vi "FTW-JSON-Core-GetFlattenedValue.vi"(0 "Container":refnum<class "FTW-Container.lvclass">, 7 "LabVIEW Type":T1, 9 "Element Default Value":variant, 11 "error in":errorcluster, 12 "Encoding Flags":i64 format="%016x") -> (4 "Flattened Value":string, 15 "error out":errorcluster)   [LabVIEW 2015]
uses:
  Reflection/FTW-Reflection-Types.ctl
  container/FTW-Container.lvclass
  Error/FTW-ERR-ThrowError.vi
panel:
  # "Inputs"
  # "Outputs"
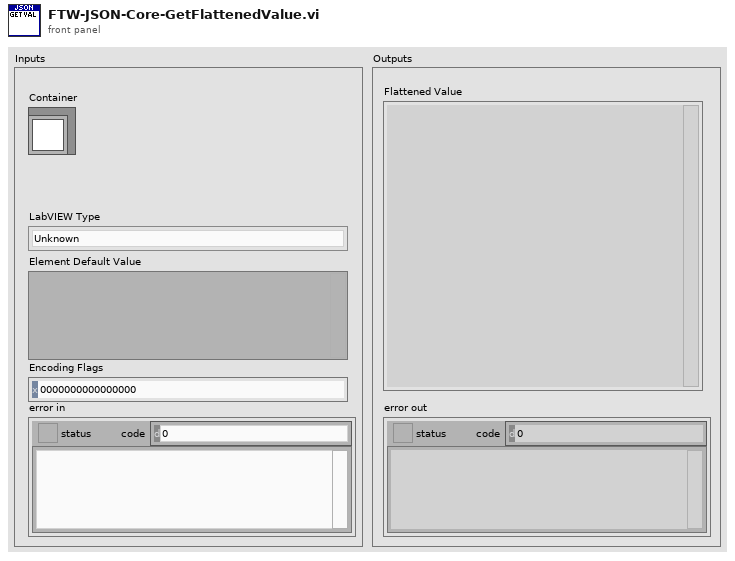
[diagram p1: front panel]
types:
  T1 = typedef "FTW-Reflection-Types.ctl" = enum16{"Unknown", "Void", "Array", "Cluster", "LVObject", "Boolean", "I8", "I16", "I32", "I64", "U8", "U16", "U32", "U64", "SGL", "DBL", "EXT", "CSG", "CDB", "CXT", "FXP", "EnumU8", "EnumU16", "EnumU32", "EnumU64", "SGLwithUnit", "DBLwithUnit", "EXTwithUnit", "CSGwithUnit", "CDBwithUnit", "CXTwithUnit", "String", "Path", "Picture", "Tag", "LVVariant", "Timestamp", "WaveformI8", "WaveformI16", "WaveformI32", "WaveformI64", "WaveformU8", "WaveformU16", "WaveformU32", "WaveformU64", "WaveformSGL", "WaveformDBL", "WaveformEXT", "WaveformCSG", "WaveformCDB", "WaveformCXT", "WaveformDigital", "WaveformUnknownType", "DigitalData", "DynamicData", "ExternalData", "FileByteStream", "TDMStream", "dotNET", "ActiveX", "VIServerReference", "VIReference", "ApplicationInstance", "Menu", "ConnectionDataSocket", "ConnectionVISA", "ConnectionBluetooth", "ConnectionIrDA", "ConnectionTCP", "ConnectionUDP", "ConnectionHTTPClient", "ConnectionFTP", "Occurrence", "Notifier", "Queue", "Rendezvous", "Semaphore", "RTFIFO", "EventPublisher", "EventRegistration", "EventCallback", "DataValueReference", "GenericClass", "GenericClassTag", "GenericClassDeepCopy", "GenericClassFlattened", "GenericClassTagFlattened", "GenericReferenceType", "WindowsRegistry", "OverloadedDatalogRef", "ReferenceUnknownType"}
  T2 = typedef "NI_Data Type.lvlib/Data Type.ctl" = enum8{"Invalid Type", "Void", "I8", "I16", "I32", "I64", "U8", "U16", "U32", "U64", "Single Float", "Double Float", "Extended Float", "Single Complex", "Double Complex", "Extended Complex", "Enum U8", "Enum U16", "Enum U32", "Enum U64", "Single Float With Unit", "Double Float With Unit", "Extended Float With Unit", "Single Complex with Unit", "Double Complex with Unit", "Extended Complex with Unit", "Boolean", "String", "Path", "Picture", "Tag", "Array", "Cluster", "Variant", "LV Variant", "Waveform", "Timestamp", "Digital Waveform", "Digital Data", "ExpressData", "Refnum", "External Data", "VI", "Poly VI", "LabVIEW Class Instance", "Fixed Point"}
  T3 = cluster{"Element Name":string, "Element Type":T1, "Element Value":variant}[]
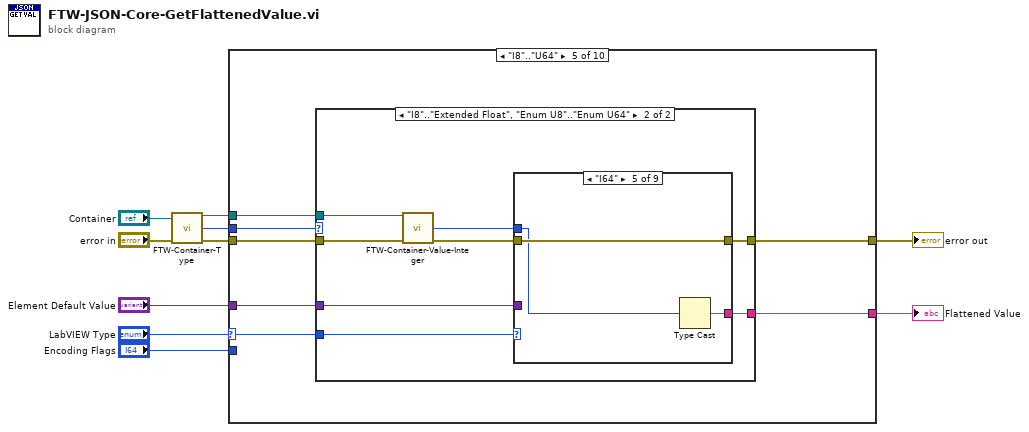
[diagram p0: block diagram]
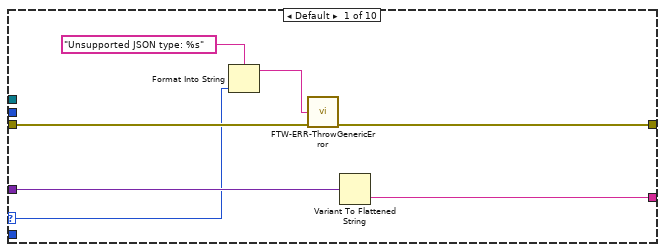
[diagram p2: hidden frame]
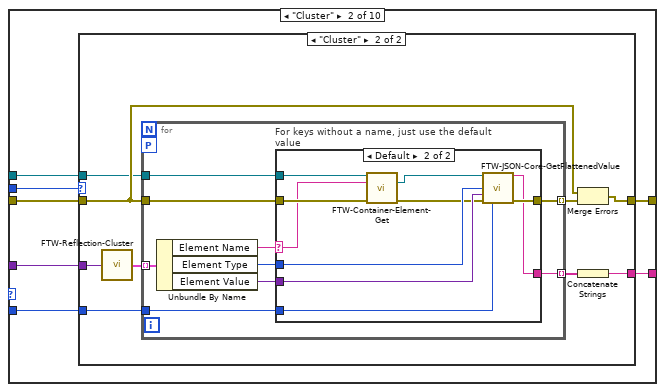
[diagram p3: hidden frame]
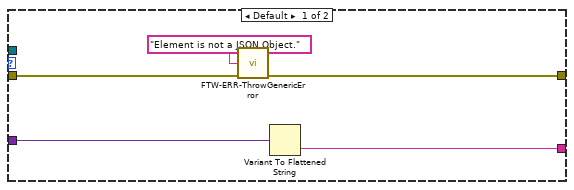
[diagram p4: hidden frame]
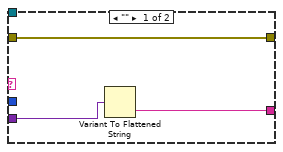
[diagram p5: hidden frame]
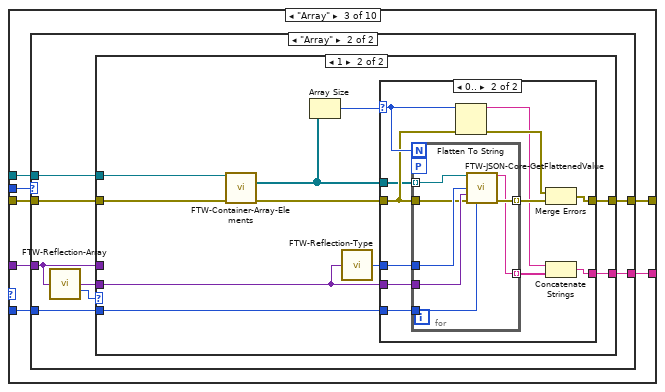
[diagram p6: hidden frame]
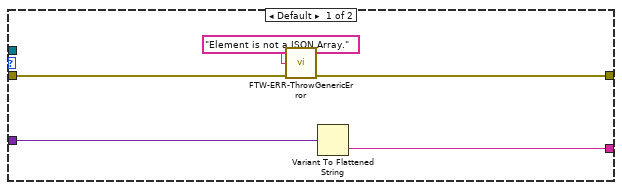
[diagram p7: hidden frame]
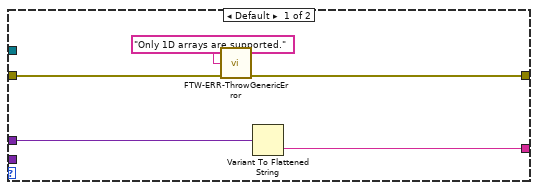
[diagram p8: hidden frame]
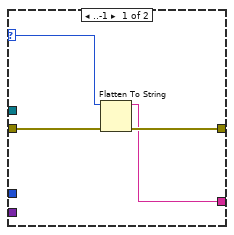
[diagram p9: hidden frame]
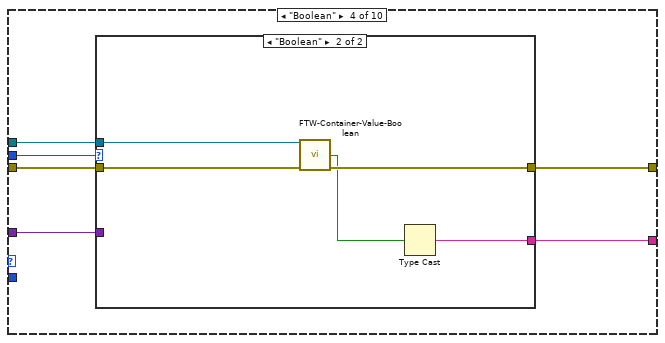
[diagram p10: hidden frame]
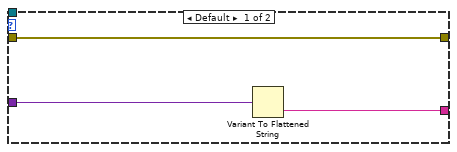
[diagram p11: hidden frame]
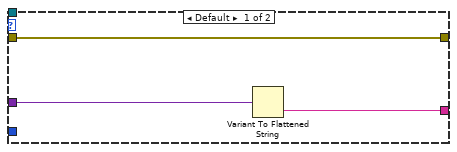
[diagram p12: hidden frame]
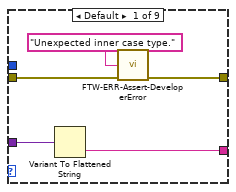
[diagram p13: hidden frame]
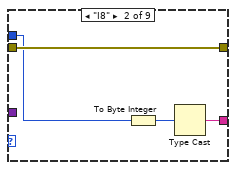
[diagram p14: hidden frame]
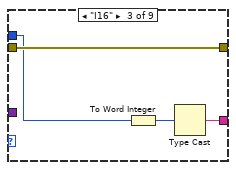
[diagram p15: hidden frame]
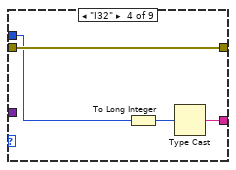
[diagram p16: hidden frame]
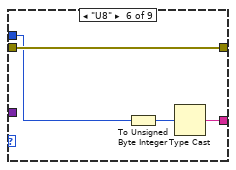
[diagram p17: hidden frame]
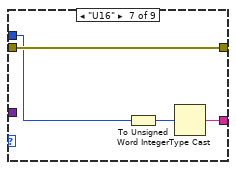
[diagram p18: hidden frame]
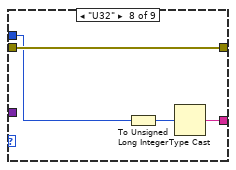
[diagram p19: hidden frame]
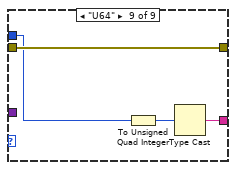
[diagram p20: hidden frame]
diagram:
  n1 = call "FTW-Container-Type.vi"("FTW-Container In"="Container", "error in"="error in") -> ("FTW-Container Out"=w2:refnum<class "FTW-Container.lvclass">, "Type"=w1:T2, "error out"=w4:errorcluster)  [unwired: 11 in]
  n2 = case shown="\"I8\"..\"U64\"" "LabVIEW Type" {
    selector: "LabVIEW Type" -> [w11 _ _ _ w136 w190 w260 _ w319 _]
    tunnel: [w14 w22 w65 w120 w134 w188 w258 w292 w317 w363] -> w10
    tunnel: [w12 w23 w66 w123 w138 w192 w262 w295 w321 w366] -> w8
    tunnel: w4 -> [w15 w21 w64 w124 w139 w193 w263 w296 w322 w367]
    tunnel: "Element Default Value" -> [w13 w24 w67 w122 w137 w191 w261 w294 w320 w365]
    tunnel: w1 -> [_ w20 w63 w121 w135 w189 w259 w293 w318 w364]
    tunnel: "Encoding Flags" -> [_ w19 w62 _ _ _ _ _ w316 _]
    tunnel: w2 -> [_ w18 w61 w119 w133 w187 w257 w291 w315 w362]
    frame Default {
      n3 = Format Into String(format string="Unsupported JSON type: %s", w11) -> (resulting string=w17:string)  [unwired: 2 in, 1 out]
      n4 = call "FTW-ERR-ThrowGenericError.vi"("Error Message"=w17, "error in"=w15) -> ("error out"=w14:errorcluster)  [unwired: 13 in]
      n5 = Variant To Flattened String(Variant=w13) -> (data string=w12:string)  [unwired: 1 out]
    }
    frame "Cluster" {
      n6 = case shown="\"Cluster\"" w20 {
        tunnel: w24 -> [w27 w38]
        tunnel: [w26 w37] -> w23
        tunnel: [w28 w36] -> w22
        tunnel: w21 -> [w29 w31]
        tunnel: w19 -> [_ w35]
        tunnel: w18 -> [_ w30]
        frame Default {
          n7 = call "FTW-ERR-ThrowGenericError.vi"("Error Message"="Element is not a JSON Object.", "error in"=w29) -> ("error out"=w28:errorcluster)  [unwired: 13 in]
          n8 = Variant To Flattened String(Variant=w27) -> (data string=w26:string)  [unwired: 1 out]
        }
        frame "Cluster" {
          n9 = call "FTW-Reflection-Cluster.vi"("Cluster"=w38) -> ("Cluster Elements"=w34:T3)  [unwired: 14 in]
          n10 = for {
            tunnel: w34 -> [w46] mode=indexing
            tunnel: [w44] -> w33 mode=indexing
            tunnel: w31 -> [w47]
            tunnel: [w42] -> w32 mode=indexing
            workers-P: _ -> [_]
            tunnel: w35 -> [w41]
            tunnel: w30 -> [w39]
            n11 = Unbundle By Name(w46) -> ("Element Name"=w40:string, "Element Type"=w43:T1, "Element Value"=w45:variant)
            n12 = case "For keys without a name, just use the default value" shown="Default" w40 {
              selector: w40 -> [_ w52]
              tunnel: w47 -> [w48 w60]
              tunnel: w45 -> [w50 w57]
              tunnel: [w49 w58] -> w44
              tunnel: w43 -> [_ w56]
              tunnel: [w48 w59] -> w42
              tunnel: w41 -> [_ w55]
              tunnel: w39 -> [_ w53]
              frame "" {
                n13 = Variant To Flattened String(Variant=w50) -> (data string=w49:string)  [unwired: 1 out]
              }
              frame Default {
                n14 = call "FTW-Container-Element-Get.vi"("FTW-Container In"=w53, "Element Name"=w52, "error in"=w60) -> ("Element Out"=w51:refnum<class "FTW-Container.lvclass">, "error out"=w54:errorcluster)  [unwired: 9 in, 2 out]
                n15 = call "FTW-JSON-Core-GetFlattenedValue.vi"("Container"=w51, "LabVIEW Type"=w56, "Element Default Value"=w57, "error in"=w54, "Encoding Flags"=w55) -> ("Flattened Value"=w58:string, "error out"=w59:errorcluster)  [unwired: 9 in]
              }
            }
          }
          n16 = Merge Errors(w31, w32) -> (w36:errorcluster)
          n17 = Concatenate Strings(w33) -> (w37:string)
        }
      }
    }
    frame "Array" {
      n18 = case shown="\"Array\"" w63 {
        tunnel: w67 -> [w70 w75]
        tunnel: [w69 w80] -> w66
        tunnel: [w68 w79] -> w65
        tunnel: w64 -> [w71 w78]
        tunnel: w62 -> [_ w74]
        tunnel: w61 -> [_ w73]
        frame Default {
          n19 = call "FTW-ERR-ThrowGenericError.vi"("Error Message"="Element is not a JSON Array.", "error in"=w71) -> ("error out"=w68:errorcluster)  [unwired: 13 in]
          n20 = Variant To Flattened String(Variant=w70) -> (data string=w69:string)  [unwired: 1 out]
        }
        frame "Array" {
          n21 = call "FTW-Reflection-Array.vi"("Array"=w75) -> ("Default Array Element"=w77:variant, "Number of Dimensions"=w76:i32)  [unwired: 13 in]
          n22 = case shown="1" w76 {
            tunnel: [w82 w95] -> w80
            tunnel: [w83 w94] -> w79
            tunnel: w78 -> [w84 w91]
            tunnel: w77 -> [_ w90]
            tunnel: w75 -> [w81 _]
            tunnel: w74 -> [_ w92]
            tunnel: w73 -> [_ w88]
            frame Default {
              n23 = call "FTW-ERR-ThrowGenericError.vi"("Error Message"="Only 1D arrays are supported.", "error in"=w84) -> ("error out"=w83:errorcluster)  [unwired: 13 in]
              n24 = Variant To Flattened String(Variant=w81) -> (data string=w82:string)  [unwired: 1 out]
            }
            frame 1 {
              n25 = call "FTW-Container-Array-Elements.vi"("FTW-Container In"=w88, "error in"=w91) -> ("Array Elements"=w86:refnum<class "FTW-Container.lvclass">[], "error out"=w89:errorcluster)  [unwired: 11 in, 1 out]
              n26 = Array Size(array=w86) -> (size(s)=w87:i32)
              n27 = call "FTW-Reflection-Type.vi"("Anything"=w90) -> ("LabVIEW Type"=w93:T1)  [unwired: 12 in, 2 out]
              n28 = case shown="0.." w87 {
                selector: w87 -> [w97 w105]
                tunnel: [w96 w111] -> w95
                tunnel: [w98 w110] -> w94
                tunnel: w89 -> [w99 w102]
                tunnel: w93 -> [_ w108]
                tunnel: w90 -> [_ w107]
                tunnel: w92 -> [_ w101]
                tunnel: w86 -> [_ w100]
                frame ..-1 {
                  n29 = Flatten To String(anything=w97, error in (no error)=w99) -> (data string=w96:string, error out=w98:errorcluster)  [unwired: 2 in, 1 out]
                }
                frame 0.. {
                  n30 = for {
                    N: w105 -> [_]
                    workers-P: _ -> [_]
                    tunnel: w102 -> [w113]
                    tunnel: [w118] -> w109 mode=indexing
                    tunnel: w108 -> [w115]
                    tunnel: w107 -> [w116]
                    tunnel: [w117] -> w106 mode=indexing
                    tunnel: w101 -> [w114]
                    tunnel: w100 -> [w112] mode=indexing
                    n31 = call "FTW-JSON-Core-GetFlattenedValue.vi"("Container"=w112, "LabVIEW Type"=w115, "Element Default Value"=w116, "error in"=w113, "Encoding Flags"=w114) -> ("Flattened Value"=w117:string, "error out"=w118:errorcluster)  [unwired: 9 in]
                  }
                  n32 = Flatten To String(anything=w105, error in (no error)=w102) -> (data string=w103:string, error out=w104:errorcluster)  [unwired: 2 in, 1 out]
                  n33 = Merge Errors(w104, w109) -> (w110:errorcluster)
                  n34 = Concatenate Strings(w103, w106) -> (w111:string)
                }
              }
            }
          }
        }
      }
    }
    frame "Boolean" {
      n35 = case shown="\"Boolean\"" w121 {
        tunnel: w124 -> [w125 w131]
        tunnel: w122 -> [w127 _]
        tunnel: [w126 w132] -> w123
        tunnel: [w125 w130] -> w120
        tunnel: w119 -> [_ w129]
        frame Default {
          n36 = Variant To Flattened String(Variant=w127) -> (data string=w126:string)  [unwired: 1 out]
        }
        frame "Boolean" {
          n37 = call "FTW-Container-Value-Boolean.vi"("FTW-Container In"=w129, "error in"=w131) -> ("Value"=w128:bool, "error out"=w130:errorcluster)  [unwired: 11 in, 1 out]
          n38 = Type Cast(x=w128) -> (*(type *) &x=w132:string)  [unwired: 1 in]
        }
      }
    }
    frame "I8".."U64" {
      n39 = case shown="\"I8\"..\"Extended Float\", \"Enum U8\"..\"Enum U64\"" w135 {
        tunnel: w139 -> [w140 w148]
        tunnel: w137 -> [w142 w146]
        tunnel: [w141 w147] -> w138
        tunnel: [w140 w149] -> w134
        tunnel: w136 -> [_ w150]
        tunnel: w133 -> [_ w144]
        frame Default {
          n40 = Variant To Flattened String(Variant=w142) -> (data string=w141:string)  [unwired: 1 out]
        }
        frame "I8".."Extended Float", "Enum U8".."Enum U64" {
          n41 = call "FTW-Container-Value-Integer.vi"("JSON"=w144, "error in"=w148) -> ("Value"=w143:i64, "error out"=w145:errorcluster)  [unwired: 11 in, 1 out]
          n42 = case shown="\"I64\"" w150 {
            tunnel: [w154 w159 w163 w167 w170 w174 w178 w182 w186] -> w149
            tunnel: w145 -> [w155 w159 w163 w167 w170 w174 w178 w182 w186]
            tunnel: w143 -> [_ w157 w161 w165 w168 w172 w176 w180 w184]
            tunnel: [w151 w158 w162 w166 w169 w173 w177 w181 w185] -> w147
            tunnel: w146 -> [w152 _ _ _ _ _ _ _ _]
            frame Default {
              n43 = Variant To Flattened String(Variant=w152) -> (data string=w151:string)  [unwired: 1 out]
              n44 = call "FTW-ERR-Assert-DeveloperError.vi"("Reason this error should never happen"="Unexpected inner case type.", "error in"=w155) -> ("error out"=w154:errorcluster)  [unwired: 13 in]
            }
            frame "I8" {
              n45 = To Byte Integer(number=w157) -> (8bit integer=w156:i8)
              n46 = Type Cast(x=w156) -> (*(type *) &x=w158:string)  [unwired: 1 in]
            }
            frame "I16" {
              n47 = To Word Integer(number=w161) -> (16bit integer=w160:i16)
              n48 = Type Cast(x=w160) -> (*(type *) &x=w162:string)  [unwired: 1 in]
            }
            frame "I32" {
              n49 = To Long Integer(number=w165) -> (32bit integer=w164:i32)
              n50 = Type Cast(x=w164) -> (*(type *) &x=w166:string)  [unwired: 1 in]
            }
            frame "I64" {
              n51 = Type Cast(x=w168) -> (*(type *) &x=w169:string)  [unwired: 1 in]
            }
            frame "U8" {
              n52 = To Unsigned Byte Integer(number=w172) -> (unsigned 8bit integer=w171:u8)
              n53 = Type Cast(x=w171) -> (*(type *) &x=w173:string)  [unwired: 1 in]
            }
            frame "U16" {
              n54 = To Unsigned Word Integer(number=w176) -> (unsigned 16bit integer=w175:u16)
              n55 = Type Cast(x=w175) -> (*(type *) &x=w177:string)  [unwired: 1 in]
            }
            frame "U32" {
              n56 = To Unsigned Long Integer(number=w180) -> (unsigned 32bit integer=w179:u32)
              n57 = Type Cast(x=w179) -> (*(type *) &x=w181:string)  [unwired: 1 in]
            }
            frame "U64" {
              n58 = To Unsigned Quad Integer(1:w184) -> (0:w183:u64)
              n59 = Type Cast(x=w183) -> (*(type *) &x=w185:string)  [unwired: 1 in]
            }
          }
        }
      }
    }
    frame "EnumU8".."EnumU64" {
      n60 = case shown="\"String\"" w189 {
        tunnel: w193 -> [w194 w206 w231]
        tunnel: w191 -> [w196 w200 w235]
        tunnel: [w195 w203 w232] -> w192
        tunnel: [w194 w204 w233] -> w188
        tunnel: w190 -> [_ w205 w234]
        tunnel: w187 -> [_ w198 w229]
        frame Default {
          n61 = Variant To Flattened String(Variant=w196) -> (data string=w195:string)  [unwired: 1 out]
        }
        frame "String" {
          n62 = call "FTW-Container-Value-String.vi"("JSON"=w198, "error in"=w206) -> ("Value"=w197:string, "error out"=w199:errorcluster)  [unwired: 11 in, 1 out]
          n63 = call "FTW-Reflection-Enum.vi"("Enum"=w200) -> ("Enum Items"=w202:string[])  [unwired: 12 in, 2 out]
          n64 = Search 1D Array(1D array=w202, element=w197) -> (index of element=w201:i32)  [unwired: 1 in]
          n65 = case shown="\"EnumU8\"" w205 {
            tunnel: [w210 w215 w219 w223 w227] -> w204
            tunnel: w199 -> [w211 w215 w219 w223 w227]
            tunnel: [w208 w214 w218 w222 w226] -> w203
            tunnel: w201 -> [_ w212 w216 w220 w224]
            tunnel: w200 -> [w207 _ _ _ _]
            frame Default {
              n66 = Variant To Flattened String(Variant=w207) -> (data string=w208:string)  [unwired: 1 out]
              n67 = call "FTW-ERR-Assert-DeveloperError.vi"("Reason this error should never happen"="Unexpected inner case type.", "error in"=w211) -> ("error out"=w210:errorcluster)  [unwired: 13 in]
            }
            frame "EnumU8" {
              n68 = To Unsigned Byte Integer(number=w212) -> (unsigned 8bit integer=w213:u8)
              n69 = Type Cast(x=w213) -> (*(type *) &x=w214:string)  [unwired: 1 in]
            }
            frame "EnumU16" {
              n70 = To Unsigned Word Integer(number=w216) -> (unsigned 16bit integer=w217:u16)
              n71 = Type Cast(x=w217) -> (*(type *) &x=w218:string)  [unwired: 1 in]
            }
            frame "EnumU32" {
              n72 = To Unsigned Long Integer(number=w220) -> (unsigned 32bit integer=w221:u32)
              n73 = Type Cast(x=w221) -> (*(type *) &x=w222:string)  [unwired: 1 in]
            }
            frame "EnumU64" {
              n74 = To Unsigned Quad Integer(1:w224) -> (0:w225:u64)
              n75 = Type Cast(x=w225) -> (*(type *) &x=w226:string)  [unwired: 1 in]
            }
          }
        }
        frame "I8".."Extended Float", "Enum U8".."Enum U64" {
          n76 = call "FTW-Container-Value-Integer.vi"("JSON"=w229, "error in"=w231) -> ("Value"=w228:i64, "error out"=w230:errorcluster)  [unwired: 11 in, 1 out]
          n77 = case shown="\"EnumU8\"" w234 {
            tunnel: [w239 w244 w248 w252 w256] -> w233
            tunnel: w230 -> [w240 w244 w248 w252 w256]
            tunnel: w228 -> [_ w242 w246 w250 w254]
            tunnel: [w236 w243 w247 w251 w255] -> w232
            tunnel: w235 -> [w237 _ _ _ _]
            frame Default {
              n78 = Variant To Flattened String(Variant=w237) -> (data string=w236:string)  [unwired: 1 out]
              n79 = call "FTW-ERR-Assert-DeveloperError.vi"("Reason this error should never happen"="Unexpected inner case type.", "error in"=w240) -> ("error out"=w239:errorcluster)  [unwired: 13 in]
            }
            frame "EnumU8" {
              n80 = To Unsigned Byte Integer(number=w242) -> (unsigned 8bit integer=w241:u8)
              n81 = Type Cast(x=w241) -> (*(type *) &x=w243:string)  [unwired: 1 in]
            }
            frame "EnumU16" {
              n82 = To Unsigned Word Integer(number=w246) -> (unsigned 16bit integer=w245:u16)
              n83 = Type Cast(x=w245) -> (*(type *) &x=w247:string)  [unwired: 1 in]
            }
            frame "EnumU32" {
              n84 = To Unsigned Long Integer(number=w250) -> (unsigned 32bit integer=w249:u32)
              n85 = Type Cast(x=w249) -> (*(type *) &x=w251:string)  [unwired: 1 in]
            }
            frame "EnumU64" {
              n86 = To Unsigned Quad Integer(1:w254) -> (0:w253:u64)
              n87 = Type Cast(x=w253) -> (*(type *) &x=w255:string)  [unwired: 1 in]
            }
          }
        }
      }
    }
    frame "SGL".."EXT" {
      n88 = case shown="\"I8\"..\"Extended Float\", \"Enum U8\"..\"Enum U64\"" w259 {
        tunnel: w263 -> [w264 w270]
        tunnel: w261 -> [w266 w271]
        tunnel: [w265 w272] -> w262
        tunnel: [w264 w273] -> w258
        tunnel: w260 -> [_ w274]
        tunnel: w257 -> [_ w268]
        frame Default {
          n89 = Variant To Flattened String(Variant=w266) -> (data string=w265:string)  [unwired: 1 out]
        }
        frame "I8".."Extended Float", "Enum U8".."Enum U64" {
          n90 = call "FTW-Container-Value-EXT.vi"("JSON"=w268, "error in"=w270) -> ("Value"=w267:ext, "error out"=w269:errorcluster)  [unwired: 11 in, 1 out]
          n91 = case shown="\"EXT\"" w274 {
            tunnel: [w278 w283 w287 w290] -> w273
            tunnel: w269 -> [w279 w283 w287 w290]
            tunnel: w267 -> [_ w280 w285 w288]
            tunnel: [w275 w282 w286 w289] -> w272
            tunnel: w271 -> [w276 _ _ _]
            frame Default {
              n92 = Variant To Flattened String(Variant=w276) -> (data string=w275:string)  [unwired: 1 out]
              n93 = call "FTW-ERR-Assert-DeveloperError.vi"("Reason this error should never happen"="Unexpected inner case type.", "error in"=w279) -> ("error out"=w278:errorcluster)  [unwired: 13 in]
            }
            frame "SGL" {
              n94 = To Single Precision Float(number=w280) -> (single precision float=w281:sgl)
              n95 = Type Cast(x=w281) -> (*(type *) &x=w282:string)  [unwired: 1 in]
            }
            frame "DBL" {
              n96 = To Double Precision Float(number=w285) -> (double precision float=w284:dbl)
              n97 = Type Cast(x=w284) -> (*(type *) &x=w286:string)  [unwired: 1 in]
            }
            frame "EXT" {
              n98 = Type Cast(x=w288) -> (*(type *) &x=w289:string)  [unwired: 1 in]
            }
          }
        }
      }
    }
    frame "Timestamp" {
      n99 = case shown="\"I8\"..\"Extended Float\", \"Enum U8\"..\"Enum U64\"" w293 {
        tunnel: w296 -> [w297 w303 w314]
        tunnel: w294 -> [w299 _ _]
        tunnel: [w298 w305 w313] -> w295
        tunnel: [w297 w302 w308] -> w292
        tunnel: w291 -> [_ w301 w307]
        frame Default {
          n100 = Variant To Flattened String(Variant=w299) -> (data string=w298:string)  [unwired: 1 out]
        }
        frame "I8".."Extended Float", "Enum U8".."Enum U64" {
          n101 = call "FTW-Container-Value-EXT.vi"("JSON"=w301, "error in"=w303) -> ("Value"=w300:ext, "error out"=w302:errorcluster)  [unwired: 11 in, 1 out]
          n102 = To Time Stamp(1:w300) -> (0:w304:timestamp)
          n103 = Type Cast(x=w304) -> (*(type *) &x=w305:string)  [unwired: 1 in]
        }
        frame "String" {
          n104 = call "FTW-Container-Value-String.vi"("JSON"=w307, "error in"=w314) -> ("Value"=w306:string, "error out"=w308:errorcluster)  [unwired: 11 in, 1 out]
          n105 = Scan From String(format string="%^<%Y-%m-%dT%H:%M:%S%3uZ>T", input string=w306, default 1=timestamp(0 s since 1904-01-01) ("Time Stamp")) -> (error out=w312:errorcluster, output 1=w311:timestamp)  [unwired: 2 in, 2 out]
          n106 = call "FTW-ERR-Clear.vi"("error to snuff"=w312) -> ()  [unwired: 1 out]
          n107 = Type Cast(x=w311) -> (*(type *) &x=w313:string)  [unwired: 1 in]
        }
      }
    }
    frame "String".."Picture", "ConnectionVISA" {
      n108 = case shown="\"U32\"" w318 {
        tunnel: w322 -> [w326 w329 w335]
        tunnel: w320 -> [_ w331 w336]
        tunnel: [w328 w330 w337] -> w321
        tunnel: [w327 w329 w338] -> w317
        tunnel: w319 -> [_ _ w339]
        tunnel: w316 -> [_ _ _]
        tunnel: w315 -> [w324 _ w333]
        frame Default {
          n109 = call "FTW-JSON-Container-Serialize.vi"("Container"=w324, "error in"=w326) -> ("JSON String"=w323:string, "error out"=w325:errorcluster)  [unwired: 12 in]
          n110 = Flatten To String(anything=w323, error in (no error)=w325) -> (data string=w328:string, error out=w327:errorcluster)  [unwired: 2 in, 1 out]
        }
        frame "U32" {
          n111 = Variant To Flattened String(Variant=w331) -> (data string=w330:string)  [unwired: 1 out]
        }
        frame "String" {
          n112 = call "FTW-Container-Value-String.vi"("JSON"=w333, "error in"=w335) -> ("Value"=w332:string, "error out"=w334:errorcluster)  [unwired: 11 in, 1 out]
          n113 = case shown="\"String\"" w339 {
            tunnel: [w343 w347 w351 w356 w361] -> w338
            tunnel: w334 -> [w344 w348 w352 w357 w361]
            tunnel: w332 -> [_ w346 w350 w355 w360]
            tunnel: [w340 w345 w349 w354 w359] -> w337
            tunnel: w336 -> [w341 _ _ _ _]
            frame Default {
              n114 = Variant To Flattened String(Variant=w341) -> (data string=w340:string)  [unwired: 1 out]
              n115 = call "FTW-ERR-Assert-DeveloperError.vi"("Reason this error should never happen"="Unexpected inner case type.", "error in"=w344) -> ("error out"=w343:errorcluster)  [unwired: 13 in]
            }
            frame "String" {
              n116 = Flatten To String(anything=w346, error in (no error)=w348) -> (data string=w345:string, error out=w347:errorcluster)  [unwired: 2 in, 1 out]
            }
            frame "ConnectionVISA" {
              n117 = Flatten To String(anything=w350, error in (no error)=w352) -> (data string=w349:string, error out=w351:errorcluster)  [unwired: 2 in, 1 out]
            }
            frame "Path" {
              n118 = String To Path(string=w355) -> (path=w353:path)
              n119 = Flatten To String(anything=w353, error in (no error)=w357) -> (data string=w354:string, error out=w356:errorcluster)  [unwired: 2 in, 1 out]
            }
            frame "Picture" {
              n120 = call "FTW-STR-Encode-Base64.vi"("Input"=w360, "Direction"=enum16{"Encode", "Decode"}."Decode") -> ("Output"=w359:string)
            }
          }
        }
      }
    }
    frame "FileByteStream".."ConnectionDataSocket", "ConnectionBluetooth".."ReferenceUnknownType" {
      n121 = case shown="\"String\"" w364 {
        tunnel: w367 -> [w368 w375]
        tunnel: w365 -> [w370 w378]
        tunnel: [w369 w380] -> w366
        tunnel: [w368 w376] -> w363
        tunnel: w362 -> [_ w372]
        frame Default {
          n122 = Variant To Flattened String(Variant=w370) -> (data string=w369:string)  [unwired: 1 out]
        }
        frame "String" {
          w381 = "0x%16x"  # Reference Format
          n123 = call "FTW-Container-Value-String.vi"("JSON"=w372, "error in"=w375) -> ("Value"=w371:string, "error out"=w373:errorcluster)  [unwired: 11 in, 1 out]
          n124 = Scan From String(format string=w381, input string=w371, error in=w373, default 1=i64 0 ("default value 1")) -> (error out=w377:errorcluster, output 1=w379:i64)  [unwired: 1 in, 2 out]
          n125 = case shown="No Error" w377 {
            selector: w377 -> [w382 _]
            tunnel: [w386 w389] -> w380
            tunnel: w379 -> [w385 _]
            tunnel: w378 -> [_ w390]
            tunnel: [w382 w388] -> w376
            frame No Error {
              n126 = Type Cast(type=refnum<k0> refnum, x=w385) -> (*(type *) &x=w384:refnum<k0>)
              n127 = Type Cast(x=w384) -> (*(type *) &x=w386:string)  [unwired: 1 in]
            }
            frame Error {
              n128 = Variant To Flattened String(Variant=w390) -> (data string=w389:string)  [unwired: 1 out]
              n129 = call "FTW-ERR-ThrowGenericError.vi"("Error Message"="Unexpected reference format.") -> ("error out"=w388:errorcluster)  [unwired: 14 in]
            }
          }
        }
      }
    }
  }
  "error out" <- w10
  "Flattened Value" <- w8
